vi "VPA QC XDCR and Scale Setup.vi"(9 "DAQ Ref Cluster":T2) -> ()   [LabVIEW 2013]
uses:
  Controls/VPA QC DAQ Ref Cluster.ctl
  Controls/VPA QC Scale Communication Settings DVR.ctl
  Controls/VPA QC Scale Communication Settings.ctl
panel:
  out "Digital Scale\nRead":dbl
  in  "Digital Scale\nCommunication \nSettings":T1={"Baud"=0, "Data Bits"=0, "Stop Bits"=0, "Parity"=enum."None", "Flow Control"=enum."RTS/CTS", "VISA resource name"=""}
  in  "Cancel":bool
  in  "OK":bool
  out "XDCR 2 PSI":dbl
  out "XDCR 2 Volts":dbl
  out "XDCR 1 PSI":dbl
  out "XDCR 1 Volts":dbl
  in  "Transducer 2\nScale Factor":dbl
  in  "Transducer 1 \nScale Factor":dbl
  in  "Transducer 2\nOffset":dbl
  in  "Transducer 1\n Offset":dbl
  # "Transducer and Scale Calibration"
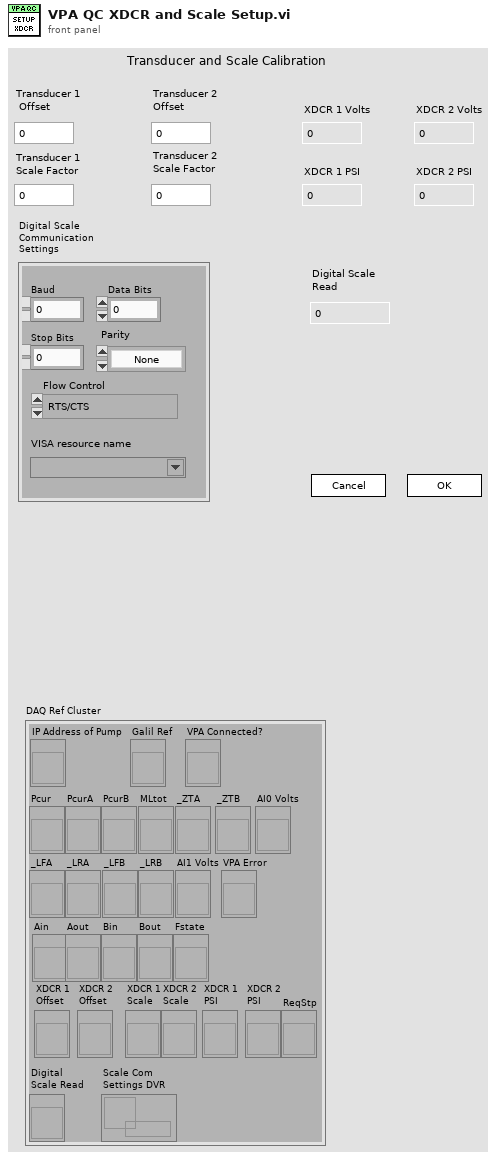
[diagram p1: front panel]
types:
  T1 = typedef "VPA QC Scale Communication Settings.ctl" = cluster{"Baud":i32, "Data Bits":i32, "Stop Bits":i32, "Parity":enum16{"None", "Odd", "Even", "Mark", "Space"}, "Flow Control":enum16{"None", "XON/XOFF", "RTS/CTS", "XON/XOFF & RTS/CTS", "DTR/DSR", "XON/XOFF & DTR/DSR"}, "VISA resource name":refnum<visa-resource-name>}
  T2 = typedef "VPA QC DAQ Ref Cluster.ctl" = cluster{"IP Address of Pump":refnum<vi>, "Galil Ref":refnum<vi>, "VPA Connected?":refnum<vi>, "Pcur":refnum<vi>, "PcurA":refnum<vi>, "PcurB":refnum<vi>, "MLtot":refnum<vi>, "_LFA":refnum<vi>, "_LRA":refnum<vi>, "_LFB":refnum<vi>, "_LRB":refnum<vi>, "_ZTA":refnum<vi>, "_ZTB":refnum<vi>, "AI0 Volts":refnum<vi>, "AI1 Volts":refnum<vi>, "VPA Error":refnum<vi>, "Ain":refnum<vi>, "Aout":refnum<vi>, "Bin":refnum<vi>, "Bout":refnum<vi>, "Fstate":refnum<vi>, "XDCR 1\nOffset":refnum<vi>, "XDCR 2 \nOffset":refnum<vi>, "XDCR 1\nScale":refnum<vi>, "XDCR 2\nScale":refnum<vi>, "XDCR 1\nPSI":refnum<vi>, "XDCR 2\nPSI":refnum<vi>, "ReqStp":refnum<vi>, "Digital \nScale Read":refnum<vi>, "Scale Com\nSettings DVR":T3}
  T3 = typedef "VPA QC Scale Communication Settings DVR.ctl" = refnum<data-value>
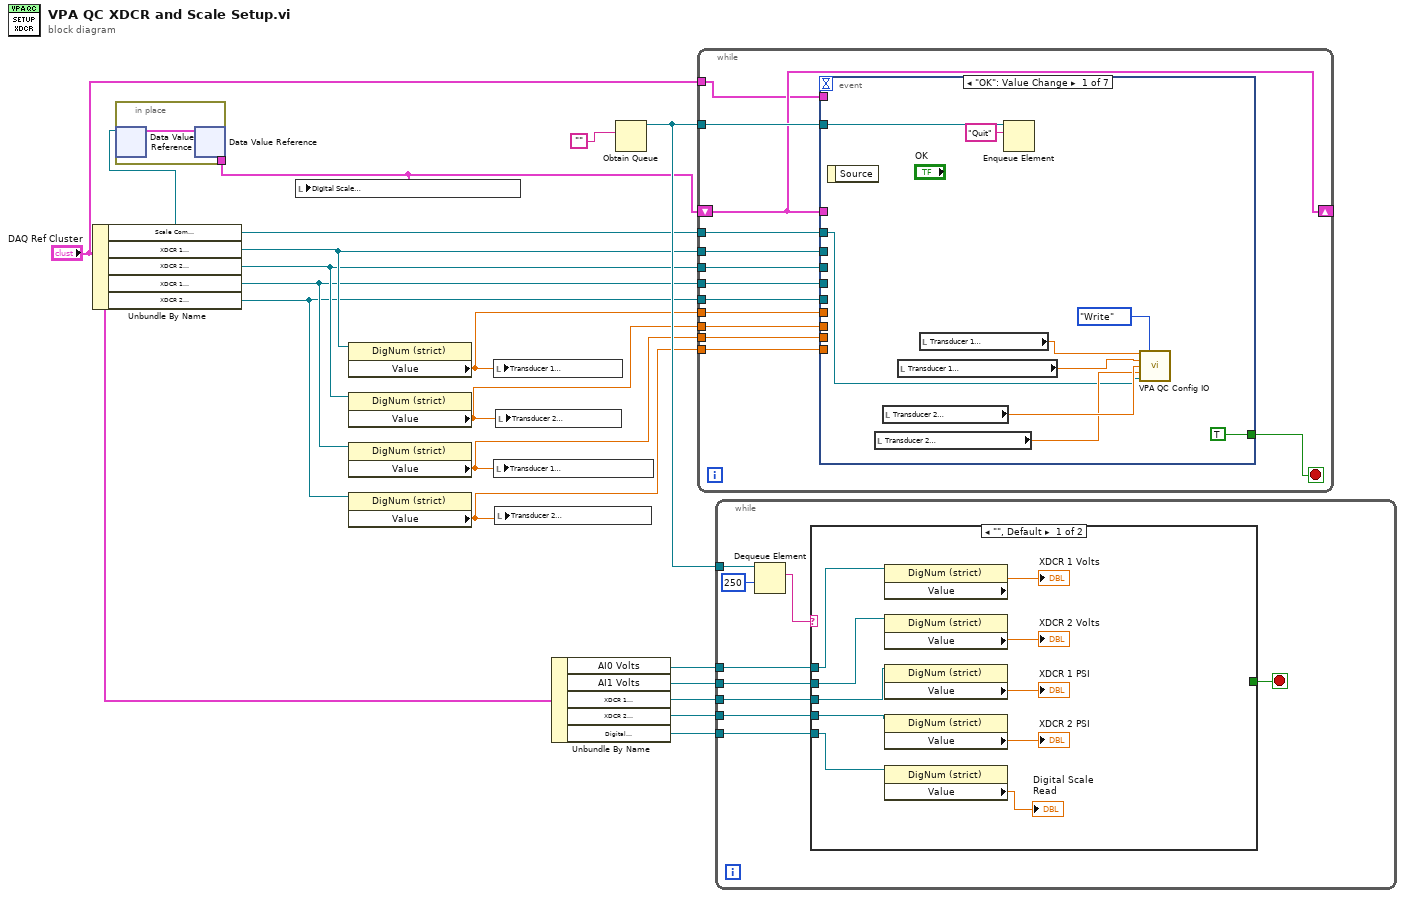
[diagram p0: block diagram]
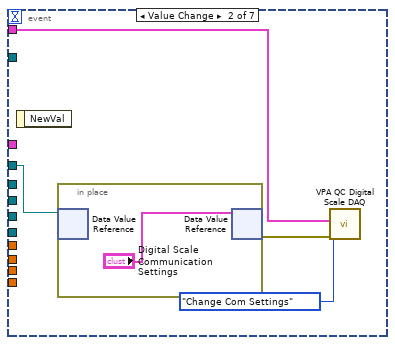
[diagram p2: hidden frame]
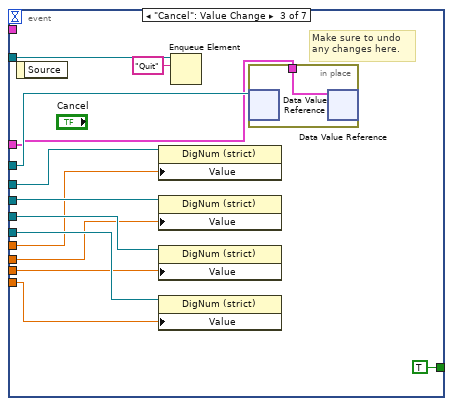
[diagram p3: hidden frame]
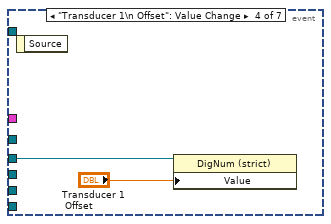
[diagram p4: hidden frame]
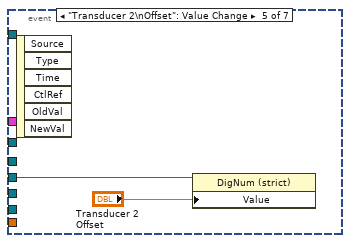
[diagram p5: hidden frame]
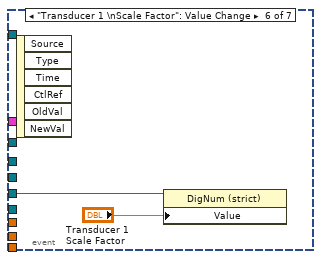
[diagram p6: hidden frame]
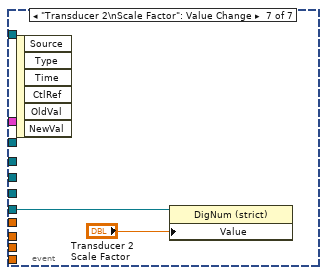
[diagram p7: hidden frame]
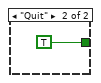
[diagram p8: hidden frame]
diagram:
  n1 = Unbundle By Name("DAQ Ref Cluster") -> ("Scale Com\nSettings DVR"=w3:T3, "XDCR 1\nOffset"=w12:refnum<vi>, "XDCR 2 \nOffset"=w11:refnum<vi>, "XDCR 1\nScale"=w10:refnum<vi>, "XDCR 2\nScale"=w9:refnum<vi>)
  n2 = in-place {
    in-place-border: [w19] -> w2
    n3 = in-place-dvr #1(w3) -> (w19:T1)  [unwired: 1 out]
    n4 = in-place-dvr #1(w19) -> ()  [unwired: 2 out]
  }
  n5 = local write "Digital Scale\nCommunication \nSettings"(w2) -> ()
  n6 = property class="DigNum (strict)"(reference=w12) -> ("Value"=w8:dbl)  [unwired: 1 in, 2 out]
  n7 = property class="DigNum (strict)"(reference=w11) -> ("Value"=w7:dbl)  [unwired: 1 in, 2 out]
  n8 = property class="DigNum (strict)"(reference=w10) -> ("Value"=w6:dbl)  [unwired: 1 in, 2 out]
  n9 = property class="DigNum (strict)"(reference=w9) -> ("Value"=w5:dbl)  [unwired: 1 in, 2 out]
  n10 = local write "Transducer 1\n Offset"(w8) -> ()
  n11 = local write "Transducer 1 \nScale Factor"(w6) -> ()
  n12 = local write "Transducer 2\nScale Factor"(w5) -> ()
  n13 = local write "Transducer 2\nOffset"(w7) -> ()
  n14 = Unbundle By Name("DAQ Ref Cluster") -> ("AI0 Volts"=w16:refnum<vi>, "AI1 Volts"=w15:refnum<vi>, "XDCR 1\nPSI"=w14:refnum<vi>, "XDCR 2\nPSI"=w13:refnum<vi>, "Digital \nScale Read"=w4:refnum<vi>)
  n15 = Obtain Queue(element data type="") -> (queue out=w17:refnum<queue>)  [unwired: 4 in, 2 out]
  n16 = while {
    tunnel: w17 -> [w27]
    tunnel: w12 -> [w31]
    tunnel: w11 -> [w30]
    tunnel: w10 -> [w29]
    tunnel: w9 -> [w28]
    tunnel: w8 -> [w26]
    tunnel: w7 -> [w25]
    tunnel: w6 -> [w23]
    tunnel: w5 -> [w24]
    tunnel: w3 -> [w22]
    shift-right: [w21] -> _
    shift-left: w2 -> [w21]
    tunnel: "DAQ Ref Cluster" -> [w20]
    stop <- w32 stop-if-true
    n17 = event shown="[0] \"OK\": Value Change" {
      selector: _ -> [_ _ _ _ _ _ _]
      dyn-events: _ -> [_ _ _ _ _ _ _]
      timeout: _ -> [_ _ _ _ _ _ _]
      tunnel: [TRUE _ TRUE _ _ _ _] -> w32
      tunnel: w31 -> [_ _ w57 w62 _ _ _]
      tunnel: w30 -> [_ _ w56 _ w64 _ _]
      tunnel: w29 -> [_ _ w55 _ _ w66 _]
      tunnel: w28 -> [_ _ w54 _ _ _ w68]
      tunnel: w27 -> [w40 _ w59 _ _ _ _]
      tunnel: w26 -> [_ _ w53 _ _ _ _]
      tunnel: w25 -> [_ _ w52 _ _ _ _]
      tunnel: w24 -> [_ _ w50 _ _ _ _]
      tunnel: w23 -> [_ _ w51 _ _ _ _]
      tunnel: w22 -> [w33 w45 w48 _ _ _ _]
      tunnel: w21 -> [_ _ w47 _ _ _ _]
      tunnel: w20 -> [_ w42 _ _ _ _ _]
      event "OK": Value Change {
        n18 = event-data() -> ()  [unwired: 1 in, 1 out]
        n19 = local read "Transducer 2\nScale Factor"() -> (w34:dbl)
        n20 = local read "Transducer 2\nOffset"() -> (w35:dbl)
        n21 = local read "Transducer 1 \nScale Factor"() -> (w36:dbl)
        n22 = local read "Transducer 1\n Offset"() -> (w37:dbl)
        n23 = Enqueue Element(queue=w40, element="Quit") -> ()  [unwired: 2 in, 3 out]
        n24 = call "VPA QC Config IO.vi"("XDCR 1 Offset"=w37, "Function"=enum16{"Read", "Write"}."Write", "XDCR 1 Scale"=w36, "XDCR 2 Offset"=w35, "XDCR 2 Scale"=w34, "DR Scale\nCom Settings In"=w33) -> ()  [unwired: 4 in, 6 out]
      }
      event Value Change {
        n25 = event-data() -> ()  [unwired: 1 in, 1 out]
        n26 = in-place {
          n27 = in-place-dvr #2(w45) -> ()  [unwired: 2 out]
          n28 = in-place-dvr #2("Digital Scale\nCommunication \nSettings") -> (w44:errorcluster)  [unwired: 1 out]
        }
        n29 = call "VPA QC Digital Scale DAQ.vi"("error in (no error)"=w44, "Function"=enum16{"Change Com Settings", "Read"}."Change Com Settings", "DAQ Ref Cluster"=w42) -> ()  [unwired: 7 in, 2 out]
      }
      event "Cancel": Value Change {
        # "Make sure to undo \nany changes here."
        n30 = event-data() -> ()  [unwired: 1 in, 1 out]
        n31 = property class="DigNum (strict)"(reference=w57, "Value"=w53) -> ()  [unwired: 1 in, 2 out]
        n32 = property class="DigNum (strict)"(reference=w56, "Value"=w52) -> ()  [unwired: 1 in, 2 out]
        n33 = property class="DigNum (strict)"(reference=w55, "Value"=w51) -> ()  [unwired: 1 in, 2 out]
        n34 = property class="DigNum (strict)"(reference=w54, "Value"=w50) -> ()  [unwired: 1 in, 2 out]
        n35 = Enqueue Element(queue=w59, element="Quit") -> ()  [unwired: 2 in, 3 out]
        n36 = in-place {
          in-place-border: w47 -> [w60]
          n37 = in-place-dvr #3(w48) -> ()  [unwired: 2 out]
          n38 = in-place-dvr #3(w60) -> ()  [unwired: 2 out]
        }
      }
      event "Transducer 1\n Offset": Value Change {
        n39 = event-data() -> ()  [unwired: 1 in, 1 out]
        n40 = property class="DigNum (strict)"(reference=w62, "Value"="Transducer 1\n Offset") -> ()  [unwired: 1 in, 2 out]
      }
      event "Transducer 2\nOffset": Value Change {
        n41 = event-data() -> ()  [unwired: 1 in, 6 out]
        n42 = property class="DigNum (strict)"(reference=w64, "Value"="Transducer 2\nOffset") -> ()  [unwired: 1 in, 2 out]
      }
      event "Transducer 1 \nScale Factor": Value Change {
        n43 = event-data() -> ()  [unwired: 1 in, 6 out]
        n44 = property class="DigNum (strict)"(reference=w66, "Value"="Transducer 1 \nScale Factor") -> ()  [unwired: 1 in, 2 out]
      }
      event "Transducer 2\nScale Factor": Value Change {
        n45 = event-data() -> ()  [unwired: 1 in, 6 out]
        n46 = property class="DigNum (strict)"(reference=w68, "Value"="Transducer 2\nScale Factor") -> ()  [unwired: 1 in, 2 out]
      }
    }
  }
  n47 = while {
    tunnel: w17 -> [w77]
    tunnel: w16 -> [w72]
    tunnel: w15 -> [w71]
    tunnel: w14 -> [w73]
    tunnel: w13 -> [w70]
    tunnel: w4 -> [w69]
    stop <- w74 stop-if-true
    n48 = Dequeue Element(queue=w77, timeout in ms (-1)=250) -> (element=w76:string)  [unwired: 1 in, 3 out]
    n49 = case shown="\"\", Default" w76 {
      tunnel: [_ TRUE] -> w74
      tunnel: w73 -> [w85 _]
      tunnel: w72 -> [w87 _]
      tunnel: w71 -> [w86 _]
      tunnel: w70 -> [w84 _]
      tunnel: w69 -> [w79 _]
      frame "", Default {
        n50 = property class="DigNum (strict)"(reference=w87) -> ("Value"=→"XDCR 1 Volts":dbl)  [unwired: 1 in, 2 out]
        n51 = property class="DigNum (strict)"(reference=w86) -> ("Value"=→"XDCR 2 Volts":dbl)  [unwired: 1 in, 2 out]
        n52 = property class="DigNum (strict)"(reference=w85) -> ("Value"=→"XDCR 1 PSI":dbl)  [unwired: 1 in, 2 out]
        n53 = property class="DigNum (strict)"(reference=w84) -> ("Value"=→"XDCR 2 PSI":dbl)  [unwired: 1 in, 2 out]
        n54 = property class="DigNum (strict)"(reference=w79) -> ("Value"=→"Digital Scale\nRead":dbl)  [unwired: 1 in, 2 out]
      }
      frame "Quit" {
      }
    }
  }
